vi "Register New Connection.vi"(8 "error in (no error)":errorcluster, 10 "TCP Connection":refnum<k5>, 11 "tWorkerController in":refnum<class "tWorkerController.lvclass">) -> (0 "error out":errorcluster, 3 "tWorkerController out":refnum<class "tWorkerController.lvclass">)   [LabVIEW 2013, in "tWorkerController.lvlib" / "tWorkerController.lvclass"]
uses:
  tWorkerController.lvclass
  <vilib>/ActorFramework/Actor/Actor.lvclass/Actor.ctl
  <vilib>/ActorFramework/Message Enqueuer/Message Enqueuer.lvclass/Message Enqueuer.ctl
  tWorkerController.lvclass/tWorkerController.ctl
  LVAutomationListener/msgs/Log Event Msg/Log Event Msg.lvclass/Log Event Msg.ctl
  _tcpConnection.ctl
  <vilib>/ActorFramework/Message Enqueuer/Message Enqueuer.lvclass
  <vilib>/ActorFramework/Message Enqueuer/Init from Existing Queue.vi
  <vilib>/ActorFramework/Message Enqueuer/Enqueue.vi
  <vilib>/ActorFramework/Message Priority Queue/Priority Enqueue.vi
  LVAutomationListener/msgs/Log Event Msg/Log Event Msg.lvclass
  tWorkerTCPConnection/tWorkerTCPConnection/tWorkerTCPConnection.lvclass
  ProcessInfo/ProcessInfo.lvlib
  <vilib>/ActorFramework/Actor/Actor.lvclass
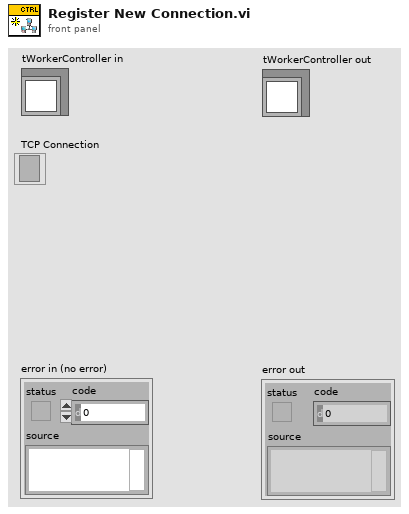
[diagram p1: front panel]
types:
  T1 = typedef "tWorkerController.lvlib/tWorkerController.lvclass/_tcpConnection.ctl" = cluster{"GUID":string, "Connection Queue":refnum<class "Message Enqueuer.lvclass">, "PID":i64}
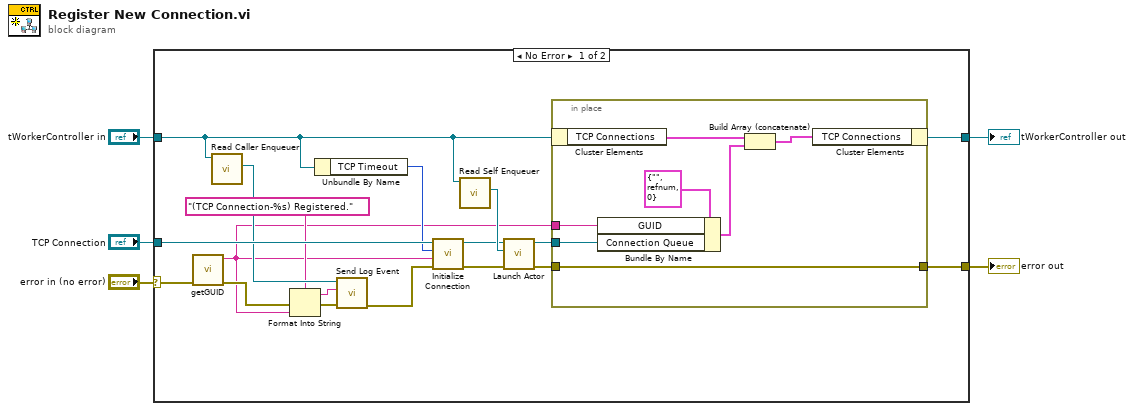
[diagram p0: block diagram]
diagram:
  n1 = case shown="No Error" "error in (no error)" {
    selector: "error in (no error)" -> [w21 w32]
    tunnel: [w15 w32] -> w4
    tunnel: [w14 w31] -> w1
    tunnel: "tWorkerController in" -> [w10 w31]
    tunnel: "TCP Connection" -> [w23 _]
    frame No Error {
      n2 = call "getGUID.vi"("error in (no error)"=w21) -> ("error out"=w12:errorcluster, "GUID"=w6:string)  [unwired: 9 in]
      n3 = call <vilib>:"Read Caller Enqueuer.vi"("Actor"=w10) -> ("Caller Enqueuer"=w9:refnum<class "Message Enqueuer.lvclass">)  [unwired: 10 in]
      n4 = Format Into String(format string="(TCP Connection-%s) Registered.", error in=w12, w6) -> (resulting string=w8:string, error out=w13:errorcluster)  [unwired: 1 in]
      n5 = Unbundle By Name(w10) -> ("TCP Timeout"=w22:i32)
      n6 = call "Send Log Event.vi"("error in (no error)"=w13, "Event Text"=w8, "Message Enqueuer"=w9) -> ("error out"=w11:errorcluster)  [unwired: 7 in, 1 out]
      n7 = call "Initialize Connection.vi"("error in (no error)"=w11, "GUID"=w6, "TCP Timeout"=w22, "TCP Connection"=w23) -> ("error out"=w18:errorcluster, "tWorkerTCPConnection out"=w19:refnum<class "tWorkerTCPConnection.lvclass">)  [unwired: 6 in]
      n8 = call <vilib>:"Read Self Enqueuer.vi"("Actor"=w10) -> ("Self Enqueuer"=w20:refnum<class "Message Enqueuer.lvclass">)  [unwired: 10 in]
      n9 = call <vilib>:"Launch Actor.vi"("error in (no error)"=w18, "Actor-to-Caller Enqueuer"=w20, "Actor"=w19) -> ("error out"=w17:errorcluster, "Caller-To-Actor Enqueuer"=w16:refnum<class "Message Enqueuer.lvclass">)  [unwired: 7 in]
      n10 = in-place {
        in-place-border: w17 -> [w25]
        in-place-border: w16 -> [w27]
        in-place-border: w6 -> [w26]
        in-place-border: [w25] -> w15
        n11 = in-place-cluster #1(w10) -> ("TCP Connections"=w30:T1[])
        n12 = Bundle By Name(cluster=T1 {"GUID"="", "Connection Queue"=refnum, "PID"=0} ("TCP Connection"), "GUID"=w26, "Connection Queue"=w27) -> (w28:T1)
        n13 = Build Array (concatenate)(w30, w28) -> (w24:T1[])
        n14 = in-place-cluster #1("TCP Connections"=w24) -> (w14:refnum<class "tWorkerController.lvclass">)
      }
    }
    frame Error {
    }
  }
  "error out" <- w4
  "tWorkerController out" <- w1
